vi "Actor Core.vi"(8 "error in":errorcluster, 11 "Red Pitaya Tester in":refnum<class "Red Pitaya Tester.lvclass">) -> (0 "error out":errorcluster, 3 "Actor out":refnum<class "Actor.lvclass">)   [LabVIEW 2015, in "Red Pitaya Tester.lvclass"]
doc: "(<B>Filename</B>: Actor Framework.lvlib:Actor.lvclass:Actor Core.vi)\n\nReceives messages to the actor, reacts to them, and initiates any error handling that may shut the actor down.\n\nDescendant classes may override this VI to append parallel tasks for the actor to complete while it handles messages. Overrides use the Call Parent Method node."
uses:
  Red Pitaya Tester.lvclass
  <vilib>/ActorFramework/Actor/Actor.lvclass
  Red Pitaya.lvclass
  Mag Lab Measure/Mag Lab Root/Mag Lab Root.lvclass/Mag Lab Root.ctl
  <vilib>/ActorFramework/Actor/Actor.lvclass/Actor.ctl
  <vilib>/ActorFramework/Message Enqueuer/Message Enqueuer.lvclass/Message Enqueuer.ctl
  <vilib>/ActorFramework/Message Enqueuer/Init from Existing Queue.vi
  <vilib>/ActorFramework/Message Enqueuer/Enqueue.vi
  <vilib>/ActorFramework/Message Priority Queue/Priority Enqueue.vi
  <vilib>/ActorFramework/Message Enqueuer/Message Enqueuer.lvclass
  <vilib>/ActorFramework/Stop Msg/Stop Msg.lvclass
  Mag Lab Measure/Mag Lab Measure Controller/Mag Lab Measure Controller.lvclass
  Mag Lab Measure/Mag Lab Root/Mag Lab Root.lvclass
panel:
  in  "Process Stop Button":bool
  in  "Play Button":bool
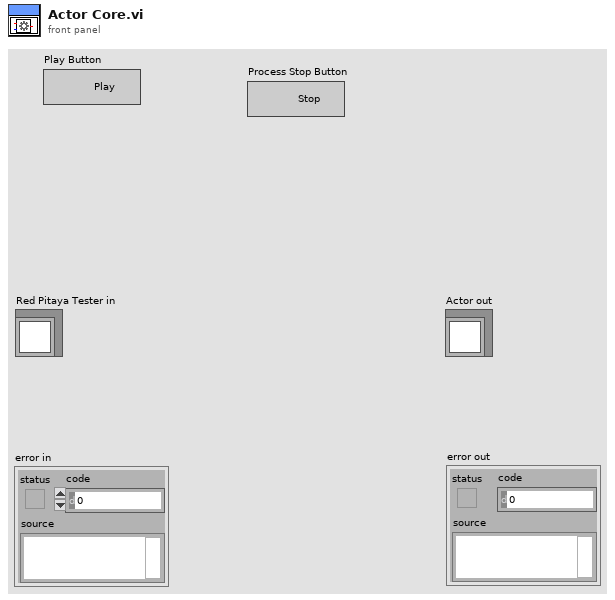
[diagram p1: front panel]
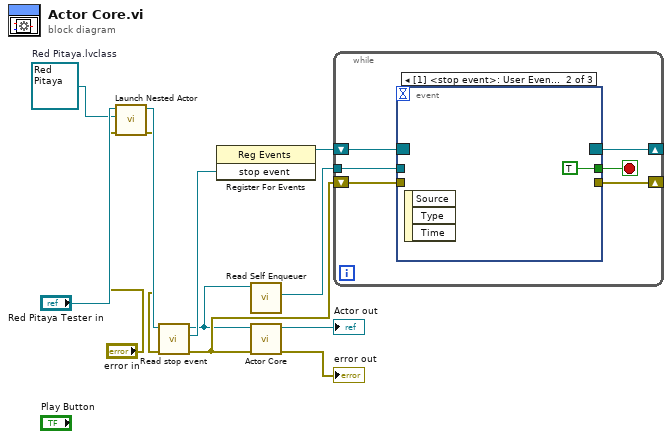
[diagram p0: block diagram]
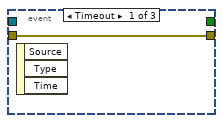
[diagram p2: hidden frame]
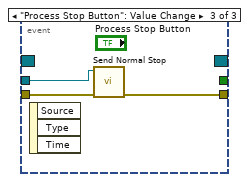
[diagram p3: hidden frame]
diagram:
  w1 = refnum<class "Red Pitaya.lvclass"> refnum  # Red Pitaya.lvclass
  n1 = call <vilib>:"Launch Nested Actor.vi"("error in (no error)"="error in", "Nested Actor"=w1, "Caller Actor in"="Red Pitaya Tester in") -> ("error out"=w2:errorcluster, "Caller Actor out"=w4:refnum<class "Red Pitaya Tester.lvclass">)  [unwired: 6 in, 1 out]
  n2 = call "Read stop event.vi"("error in (no error)"=w2, "Mag Lab Root in"=w4) -> ("error out"=w9:errorcluster, "stop event"=w10:refnum<user-event>, "Mag Lab Root out"=w7:refnum<class "Red Pitaya Tester.lvclass">)  [unwired: 7 in]
  n3 = register-events(w10) -> (reference out=w8:refnum<event-registration>)  [unwired: 2 in, 1 out]
  n4 = call <vilib>:"Read Self Enqueuer.vi"("Actor"=w7) -> ("Self Enqueuer"=w6:refnum<class "Message Enqueuer.lvclass">)  [unwired: 10 in]
  n5 = call-parent "Actor Core.vi"("error in"=w9, "Mag Lab Measure Base in"=w7) -> ("error out"=→"error out":errorcluster, "Actor out"=→"Actor out":refnum<class "Actor.lvclass">)  [unwired: 8 in]
  n6 = while {
    shift-right: [w14] -> _
    shift-left: w9 -> [w15]
    shift-right: [w17] -> _
    shift-left: w8 -> [w18]
    tunnel: w6 -> [w16]
    stop <- w13 stop-if-true
    n7 = event shown="[1] <stop event>: User Event" {
      selector: w18 -> [_ _ _]
      dyn-events: [_ _ _] -> w17
      timeout: _ -> [_ _ _]
      tunnel: w16 -> [_ _ w23]
      tunnel: w15 -> [w19 _ w22]
      tunnel: [w19 _ w21] -> w14
      tunnel: [_ TRUE _] -> w13
      event Timeout {
        n8 = event-data() -> ()  [unwired: 1 in, 3 out]
      }
      event User Event {
        n9 = event-data() -> ()  [unwired: 1 in, 3 out]
      }
      event "Process Stop Button": Value Change {
        n10 = event-data() -> ()  [unwired: 1 in, 3 out]
        n11 = call <vilib>:"Send Normal Stop.vi"("error in (no error)"=w22, "Message Enqueuer"=w23) -> ("error out"=w21:errorcluster)  [unwired: 9 in]
      }
    }
  }
